vi "sensor cmd poke.vi"(9 "new_value":u8, 10 "address":u32, 11 "device_handle":u32) -> (2 "function return":i32, 3 "device_handle out":u32)   [LabVIEW 2019, in "apdm.lvlib"]
doc: "APDM_EXPORT int apdm_sensor_cmd_poke(apdm_device_handle_t device_handle, const uint32_t address, uint8_t new_value);"
uses:
  apdm.lvlib
  Lee Lab/CP FES Walking 2018/Code/Working/LabVIEW/apdm.dll
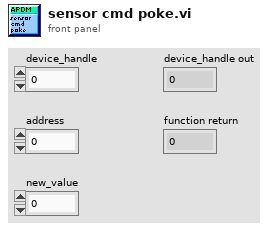
[diagram p1: front panel]
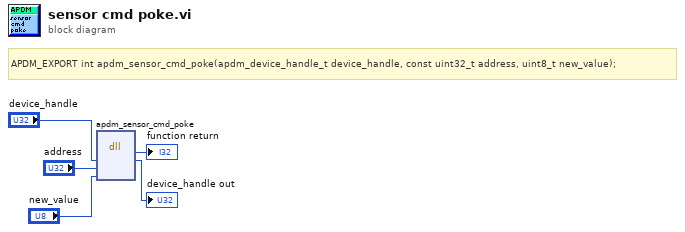
[diagram p0: block diagram]
diagram:
  # "APDM_EXPORT int apdm_sensor_cmd_poke(apdm_device_handle_t device_handle, const uint32_t address, uint8_t new_value);"
  n1 = dll-call lib="C:/Users/jfalesi/Dropbox/Lee Lab/CP FES Walking 2018/Code/Working/LabVIEW/apdm.*" fn="apdm_sensor_cmd_poke"("device_handle"="device_handle", "address"="address", "new_value"="new_value") -> (→"function return":i32, "device_handle"=→"device_handle out":u32)  [unwired: 5 in, 2 out]
